vi "target.vi"() -> ()   [LabVIEW 2018]
uses:
  <vilib>/Platform/TimedLoop/XDataNode/timing_clust.ctl
  <vilib>/Platform/TimedLoop/XDataNode/nitl_modes.ctl
  <vilib>/Platform/TimedLoop/XDataNode/wakeup.ctl
  <vilib>/rvi/Emulation/niFpgaGetClockAttributes.vi
  <vilib>/rvi/Emulation/niFpgaSctlEmulationGetInTimedLoop.vi
  <vilib>/rvi/Emulation/niFpgaEmulationReportErrorSimple.vi
  <vilib>/rvi/Emulation/niFpgaCriticalErrorInLSC.vi
  <vilib>/rvi/eio/common/nirviEmuTemplateMethod_errors.vi
  <vilib>/rvi/Emulation/niFpgaProcessEmulError.vi
  <vilib>/Platform/TimedLoop/XDataNode/XDataNode.xnode
  <vilib>/eio/EIONode/EIONode.xnode
  <vilib>/Platform/TimedLoop/XDataNode/XDNodeRunTimeDep.lvlib
panel:
  in  "PFI_WE_array":bool[](array[boolean])
  in  "SCL_array":bool[](array[boolean])
  in  "SDA_array":bool[](array[boolean])
  out "DETECT":bool=TRUE
  out "SDA_READED":u64=1
  out "SPI_READY":bool=TRUE
  in  "SPI_END":i32=49
  in  "counterLowFreq":i32=120
  in  "TEST_EEPROM":bool=TRUE
  in  "stop":bool
  in  "Start":bool
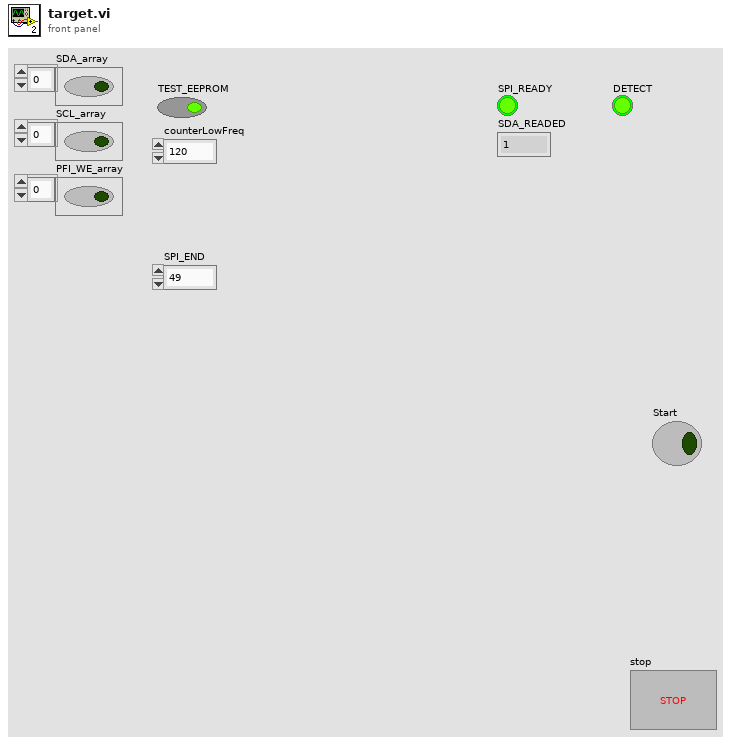
[diagram p1: front panel]
types:
  T1 = typedef "XDNodeRunTimeDep.lvlib/timing_clust.ctl" = cluster{"Expected End [f-1]":u64, "Actual End [f-1]":u64, "Finished Late? [f-1]":bool, "Expected End [i-1]":u64, "Actual End [i-1]":u64, "Finished Late? [i-1]":bool, "Expected Start [i]":u64, "Actual Start [i]":u64, "Expected Start [f]":u64, "Actual Start [f]":u64, "Source Name":string, "Structure Name":string, "Period":i64, "Deadline":i64, "Offset":i64, "Start":i64, "Priority":i32, "Timeout":i32, "Mode":T2, "Wakeup Reason":T3, "Error":errorcluster, "Source Type":string, "Secondary Source Type":string, "Global End Time":u64, "Global Start Time":u64, "Frame Duration":u64, "Iteration Duration":u64, "Assigned CPU":i32, "I/O Scan Engine Mode":u32}
  T2 = typedef "XDNodeRunTimeDep.lvlib/nitl_modes.ctl" = enum32{"No Change", "Process missed periods, maintain original phase", "Discard missed periods, maintain original phase", "Process missed periods, ignore original phase", "Discard missed periods, ignore original phase"}
  T3 = typedef "XDNodeRunTimeDep.lvlib/wakeup.ctl" = enum32{"Normal", "Aborted", "Asynchronous wakeup", "Timing source error", "Timed loop error", "Timeout"}
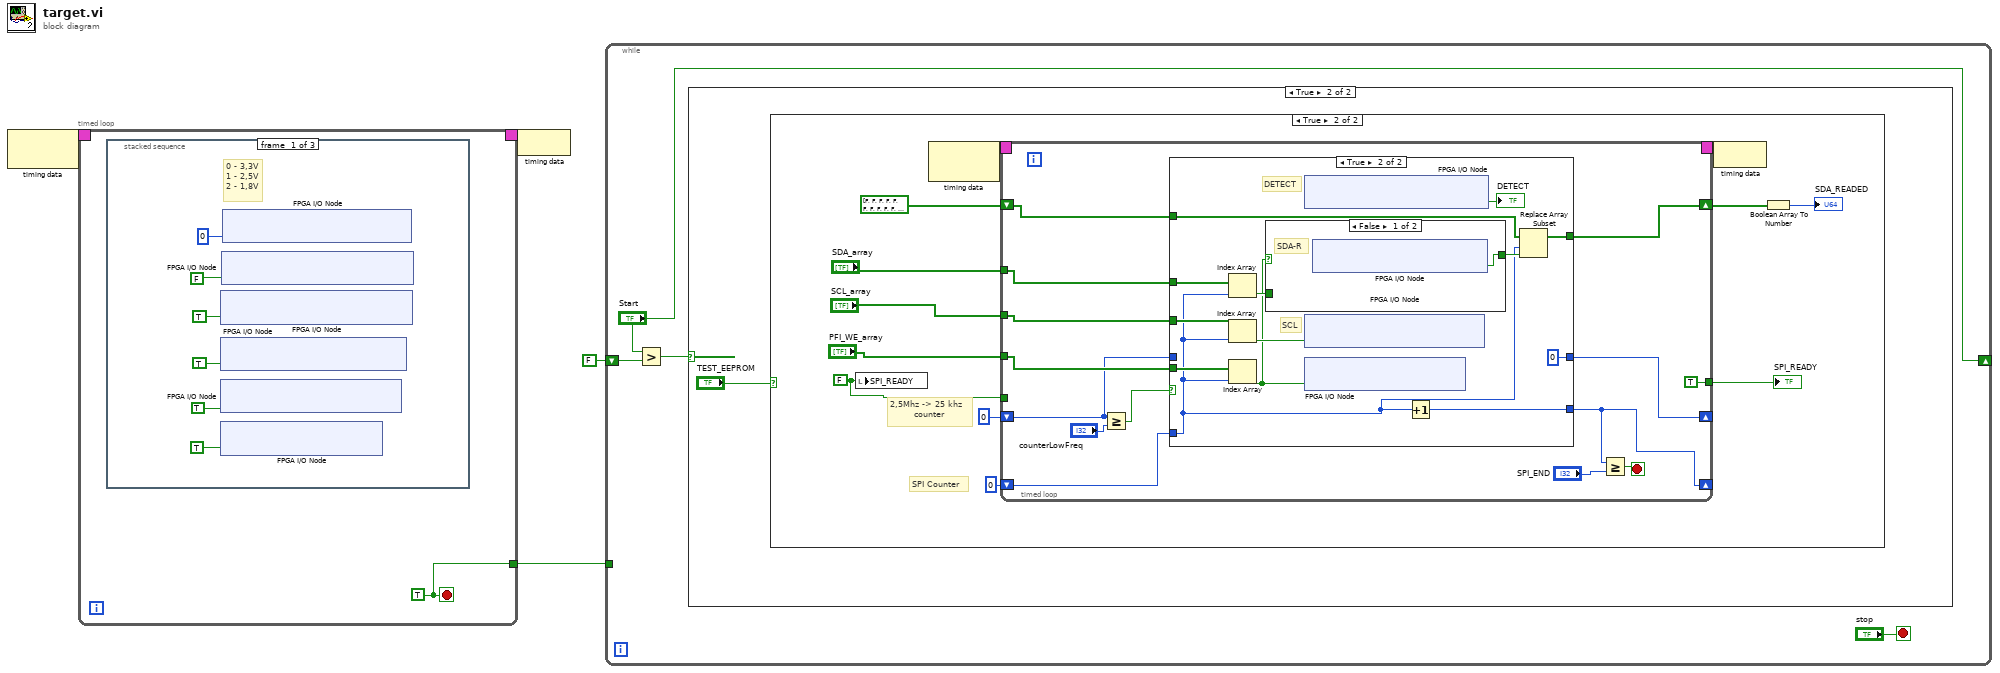
[diagram p0: block diagram]
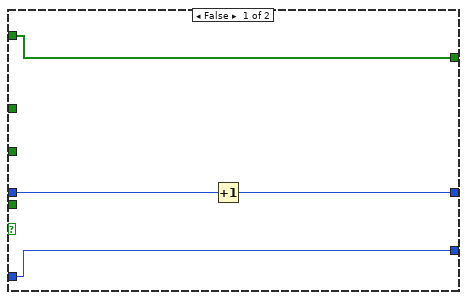
[diagram p4: hidden frame]
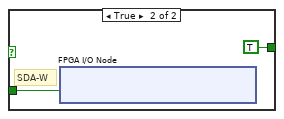
[diagram p5: hidden frame]
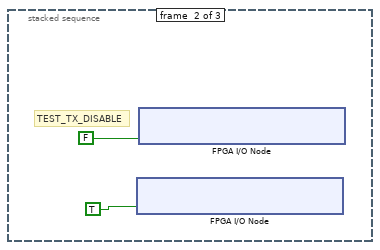
[diagram p6: hidden frame]
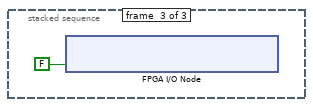
[diagram p7: hidden frame]
diagram:
  n1 = node-c288() -> (w4:T1)  [unwired: 1 in]
  n2 = timed-loop {
    timing: w4 -> [_]
    timing-out: [_] -> w3
    tunnel: [w5] -> w1
    stop <- w5 stop-if-true
    w5 = TRUE
    n3 = stacked-sequence {
      frame #0 {
        # "0 - 3,3V\n1 - 2,5V\n2 - 1,8V"
        n4 = xnode "FPGA I/O Node"("IO Module\\DDCA_DIO16-23_WE"=TRUE ("IO Module\\DDCA_DIO16-23_WE")) -> ()  [unwired: 1 in, 1 out]
        n5 = xnode "FPGA I/O Node"("IO Module\\DDCA_DIO8-15_WE"=TRUE ("IO Module\\DDCA_DIO8-15_WE")) -> ()  [unwired: 1 in, 1 out]
        n6 = xnode "FPGA I/O Node"("IO Module\\DDCA_DIO0-7_WE"=TRUE ("IO Module\\DDCA_DIO0-7_WE")) -> ()  [unwired: 1 in, 1 out]
        n7 = xnode "FPGA I/O Node"("IO Module\\DDCA_PFI_WE"=TRUE ("IO Module\\DDCA_DIO0-7_WE")) -> ()  [unwired: 1 in, 1 out]
        n8 = xnode "FPGA I/O Node"("IO Module\\DDCA_Supply_Select"=FALSE ("IO Module\\DDCA_Supply_Select")) -> ()  [unwired: 1 in, 1 out]
        n9 = xnode "FPGA I/O Node"("IO Module\\Local_Supply_Select"=u8 0 ("Local_Supply_Select")) -> ()  [unwired: 1 in, 1 out]
      }
      frame #1 {
        # "TEST_TX_DISABLE"
        n10 = xnode "FPGA I/O Node"("IO Module\\DDCA_DIO21_Write"=TRUE) -> ()  [unwired: 1 in, 1 out]
        n11 = xnode "FPGA I/O Node"("IO Module\\DDCA_DIO12_Write"=FALSE) -> ()  [unwired: 1 in, 1 out]
      }
      frame #2 {
        n12 = xnode "FPGA I/O Node"("IO Module\\DDCA_DIO16-23_WE"=FALSE ("IO Module\\DDCA_DIO16-23_WE")) -> ()  [unwired: 1 in, 1 out]
      }
    }
  }
  n13 = node-c288(w3) -> ()
  n14 = while {
    shift-right: ["Start"] -> _
    shift-left: FALSE -> [w20]
    tunnel: w1 -> [_]
    stop <- "stop" stop-if-true
    n15 = Greater?(x="Start", y=w20) -> (0:w17:bool)
    n16 = case shown="True" w17 {
      frame False {
      }
      frame True {
        n17 = case shown="True" "TEST_EEPROM" {
          frame False {
          }
          frame True {
            w25 = FALSE ("SPI_READY")
            # "2,5Mhz -> 25 khz\n        counter"
            # "SPI Counter"
            n18 = local write "SPI_READY"(w25) -> ()
            n19 = node-c288() -> (w33:T1)  [unwired: 1 in]
            n20 = timed-loop {
              timing: w33 -> [_]
              timing-out: [_] -> w32
              shift-right: [w34] -> _
              shift-left: 0 -> [w35]
              shift-right: [w36] -> _
              shift-left: 0 -> [w37]
              tunnel: "SDA_array" -> [w43]
              tunnel: "SCL_array" -> [w42]
              tunnel: "PFI_WE_array" -> [w44]
              tunnel: [TRUE] -> w26
              shift-right: [w39] -> w28
              shift-left: bool[] [FALSE, FALSE, FALSE, FALSE, FALSE, FALSE, FALSE, FALSE, FALSE, FALSE, FALSE, FALSE, FALSE, FALSE, FALSE, FALSE, FALSE, FALSE, FALSE, FALSE, FALSE, FALSE, FALSE, FALSE, FALSE, FALSE, FALSE, FALSE, FALSE, FALSE, FALSE, FALSE, FALSE, FALSE, FALSE, FALSE, FALSE, FALSE, FALSE, FALSE, FALSE, FALSE, FALSE, FALSE, FALSE, FALSE, FALSE, FALSE, FALSE, FALSE, FALSE, FALSE, FALSE, FALSE, FALSE, FALSE, FALSE, FALSE, FALSE, FALSE, FALSE, FALSE, FALSE, FALSE] -> [w40]
              tunnel: w25 -> [_]
              stop <- w47 stop-if-true
              n21 = Greater Or Equal?(x=w37, y="counterLowFreq") -> (x >= y?=w38:bool)
              n22 = case shown="True" w38 {
                tunnel: w44 -> [_ w64]
                tunnel: w43 -> [_ w62]
                tunnel: w42 -> [_ w61]
                tunnel: w40 -> [w48 w59]
                tunnel: w35 -> [w49 w52]
                tunnel: [w48 w58] -> w39
                tunnel: w37 -> [w51 _]
                tunnel: [w50 0] -> w36
                tunnel: [w49 w55] -> w34
                frame False {
                  n23 = Increment(x=w51) -> (x+1=w50:i32)
                }
                frame True {
                  # "DETECT"
                  # "SCL"
                  n24 = Index Array(array=w62, index=w52) -> (element=w63:bool)
                  n25 = Index Array(array=w61, index=w52) -> (element=w60:bool)
                  n26 = Index Array(array=w64, index=w52) -> (element=w54:bool)
                  n27 = case shown="False" w54 {
                    tunnel: w63 -> [_ w67]
                    tunnel: [w65 TRUE ("IO Module\\DDCA_PFI2_Read")] -> w53
                    frame False {
                      # "SDA-R"
                      n28 = xnode "FPGA I/O Node"() -> ("IO Module\\DDCA_PFI2_Read"=w65:bool)  [unwired: 1 in, 1 out]
                    }
                    frame True {
                      # "SDA-W"
                      n29 = xnode "FPGA I/O Node"("IO Module\\DDCA_PFI2_Write"=w67) -> ()  [unwired: 1 in, 1 out]
                    }
                  }
                  n30 = xnode "FPGA I/O Node"() -> ("IO Module\\DDCA_DIO21_Read"=→"DETECT":bool)  [unwired: 1 in, 1 out]
                  n31 = xnode "FPGA I/O Node"("IO Module\\DDCA_DIO2_Write"=w60) -> ()  [unwired: 1 in, 1 out]
                  n32 = xnode "FPGA I/O Node"("IO Module\\DDCA_PFI_WE"=w54) -> ()  [unwired: 1 in, 1 out]
                  n33 = Increment(x=w52) -> (x+1=w55:i32)
                  n34 = Replace Array Subset(array=w59, new element=w53, index=w52) -> (w58:bool[])
                }
              }
              n35 = Greater Or Equal?(x=w34, y="SPI_END") -> (x >= y?=w47:bool)
            }
            "SPI_READY" <- w26
            n36 = node-c288(w32) -> ()
            n37 = Boolean Array To Number(Boolean array=w28) -> (number=→"SDA_READED":u64)
          }
        }
      }
    }
  }
